vi "Read Current Channel.vi"(8 "error in (no error)":errorcluster, 11 "Channel Scanner Driver in":refnum<class "Channel Scanner Driver.lvclass">) -> (0 "error out":errorcluster, 2 "Current channel":i32, 3 "Channel Scanner Driver out":refnum<class "Channel Scanner Driver.lvclass">)   [LabVIEW 2019, in "Channel Scanner Driver.lvclass"]
uses:
  Channel Scanner Driver.lvclass
  Channel Scanner Driver.lvclass/Channel Scanner Driver.ctl
  Read Scan Channels.vi
  Read Next channel idx.vi
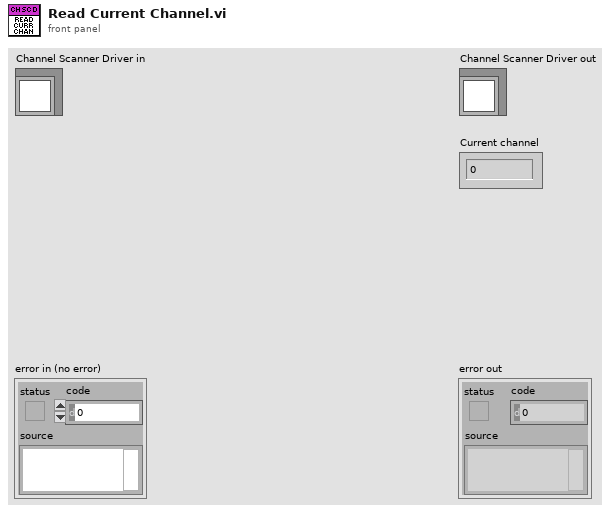
[diagram p1: front panel]
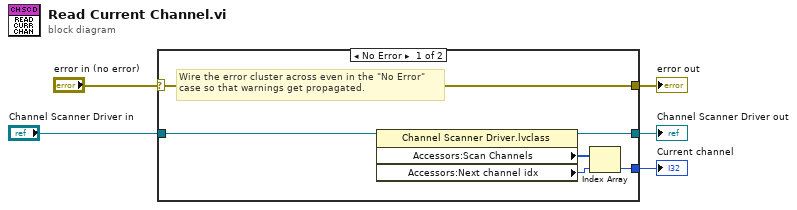
[diagram p0: block diagram]
diagram:
  n1 = case shown="No Error" "error in (no error)" {
    selector: "error in (no error)" -> [w11 w13]
    tunnel: [w11 w13] -> w4
    tunnel: [w10 w12] -> w2
    tunnel: "Channel Scanner Driver in" -> [w9 w12]
    tunnel: [w6 _] -> w1
    frame No Error {
      # "Wire the error cluster across even in the \"No Error\"\ncase so that warnings get propagated."
      n2 = property class="Channel Scanner Driver.lvclass"(reference=w9) -> (reference out=w10:refnum<class "Channel Scanner Driver.lvclass">, "Accessors:Scan Channels"=w8:i32[], "Accessors:Next channel idx"=w7:i32)  [unwired: 1 in, 1 out]
      n3 = Index Array(array=w8, index=w7) -> (element=w6:i32)
    }
    frame Error {
    }
  }
  "error out" <- w4
  "Channel Scanner Driver out" <- w2
  "Current channel" <- w1
